vi "lvProfileJSONout.vi"(3 "error in (no error)":errorcluster, 5 "Path to Python.exe":path=path "C:/ProgramData/Anaconda3/python.exe") -> (0 "error out":errorcluster, 1 "Raw Python String Output":string, 2 "Database Profiles":cluster{"profile_name":string[]})   [LabVIEW 2017]
panel:
  out "Standard Error":string
  out "Return Code":i32
  # "1. Inputs - Set before running VI"
  # "2. Outputs"
  # "3. Errors - Both Standard and LabVIEW"
  # "A + B ="
  # "This VI sends inputs to a simple Python script, and returns its output.\n\nSee block diagram for code and comments"
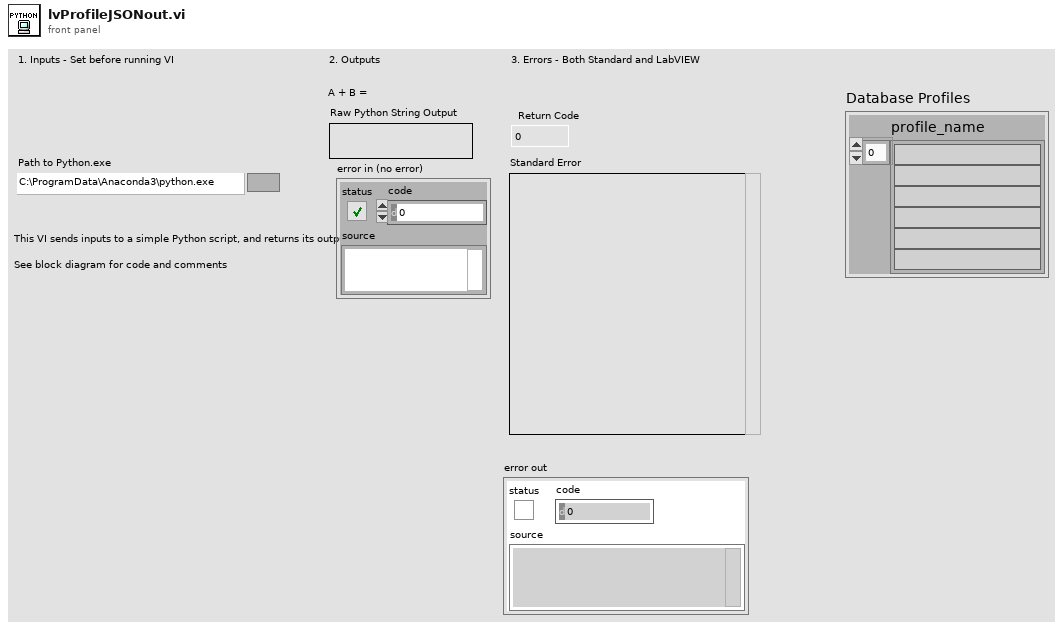
[diagram p1: front panel]
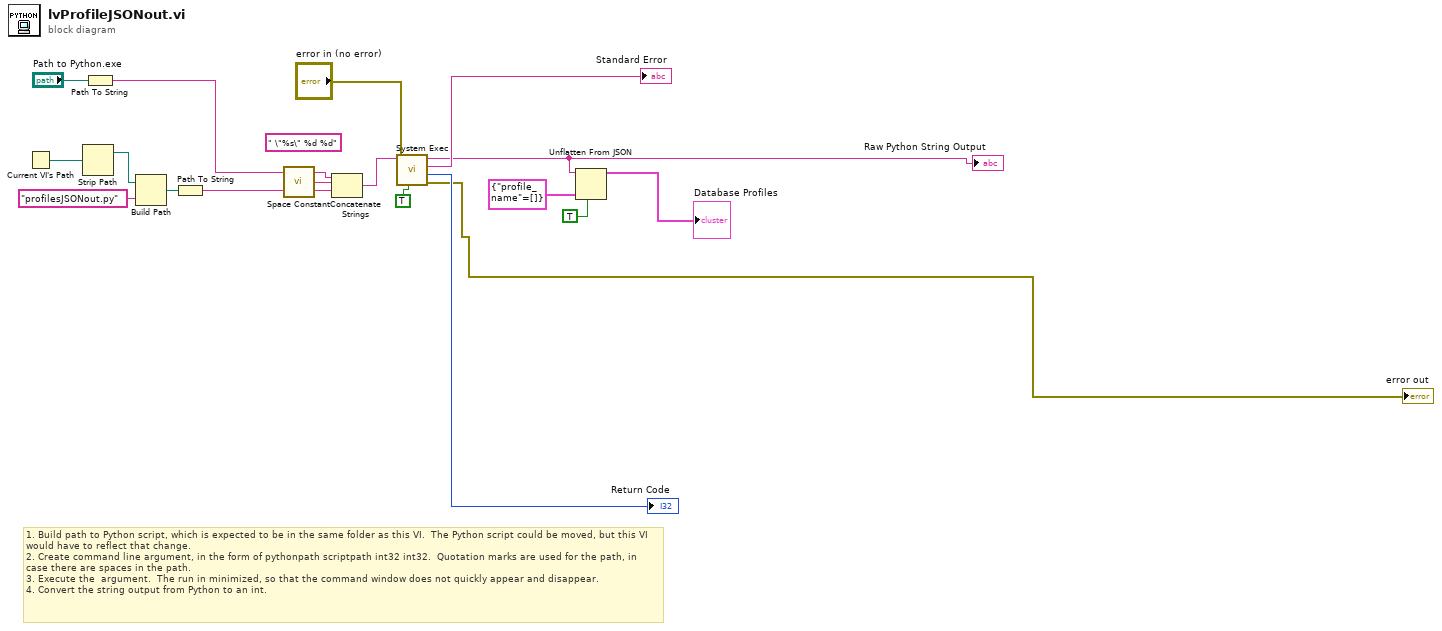
[diagram p0: block diagram]
diagram:
  (unwired) " \"%s\" %d %d" ("format string")
  # "1. Build path to Python script, which is expected to be in the same folder as this VI.  The Python script could be moved, but this VI would have to reflect that change.\n2. Create command line argument, in the form of pythonpath scriptpath int32 int32.  Quotation marks are used for the path, in case there are spaces in the path.\n3. Execute the  argument.  The run in minimized, so that the command window does not quickly appear and disappear.\n4. Convert the string output from Python to an int."
  n1 = Current VI's Path() -> (path=w13:path)
  n2 = Strip Path(path=w13) -> (stripped path=w11:path)  [unwired: 1 out]
  n3 = Path To String(path="Path to Python.exe") -> (string=w8:string)
  n4 = Build Path(base path=w11, name or relative path="profilesJSONout.py" ("Path to Function")) -> (appended path=w14:path)
  n5 = Path To String(path=w14) -> (string=w9:string)
  n6 = call <vilib>:"Space Constant.vi"() -> ("String"=w6:string)
  n7 = Concatenate Strings(w8, w6, w9) -> (w10:string)
  n8 = call <vilib>:"System Exec.vi"("run minimized? (F)"=TRUE, "error in (no error)"="error in (no error)", "command line"=w10) -> ("error out"=→"error out":errorcluster, "return code"=→"Return Code":i32, "standard error"=→"Standard Error":string, "standard output"=w3:string)  [unwired: 5 in]
  "Raw Python String Output" <- w3
  n9 = Unflatten From JSON(JSON string=w3, type and defaults=cluster{"profile_name":string[]} {"profile_name"=[]}, default null elements? (F)=TRUE) -> (value=→"Database Profiles":cluster{"profile_name":string[]})  [unwired: 4 in, 1 out]
